vi "HSD_RELAY CONTROL.vi"(8 "error in (no error)":errorcluster, 9 "State":T1 items=["0"=0, "1"=1, "X"=5], 10 "Function":T2=1100 items=["Digital"=1100, "PPMU"=1101, "Off"=1102, "Disconnect"=1103], 11 "Digital SSC in":T3[](array[typedef])) -> (0 "error out":errorcluster)   [LabVIEW 2019]
uses:
  Instrument Control/Digital/SSC Digital/SSC Digital.ctl
  <instrlib>/niDigital/niDigital.llb/niDigital Selected Function.ctl
  <instrlib>/niDigital/niDigital.llb/niDigital Write Static Pin State.ctl
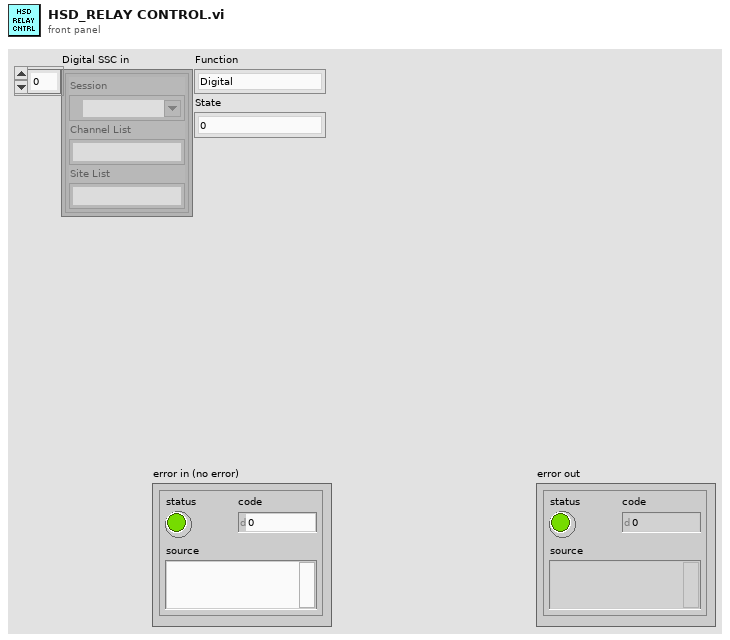
[diagram p1: front panel]
types:
  T1 = typedef "niDigital Write Static Pin State.ctl" = u8
  T2 = typedef "niDigital Selected Function.ctl" = i32
  T3 = typedef "SSC Digital.ctl" = cluster{"Session":refnum<k15>, "Channel List":string, "Site List":string}
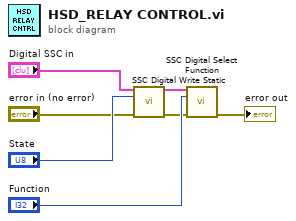
[diagram p0: block diagram]
diagram:
  n1 = call "SSC Digital Write Static.vi"("Digital SSC in"="Digital SSC in", "State"="State", "error in"="error in (no error)") -> ("Digital SSC out"=w3:T3[], "error out"=w2:errorcluster)  [unwired: 11 in]
  n2 = call "SSC Digital Select Function.vi"("Digital SSC in"=w3, "Function"="Function", "error in"=w2) -> ("error out"=→"error out":errorcluster)  [unwired: 11 in, 1 out]
